vi "Aurdino Mode Lights.vi"(0 "Climb":bool, 7 "Tracks Down":bool, 8 "Robot Centric":bool, 9 "Field Centric":bool) -> ()   [LabVIEW 2017]
uses:
  <vilib>/Rock Robotics/Network Tables/NT Read Boolean.vi
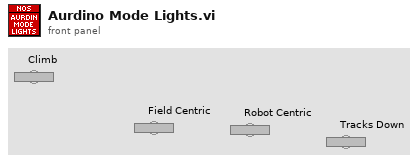
[diagram p1: front panel]
types:
  T1 = typedef "WPI_DigitalInputDevRef.ctl" = cluster{"DevStatus":errorcluster, "DIO Channel":T2}
  T2 = typedef "FPGA_DIOChannel.ctl" = enum8{"DIO 0", "DIO 1", "DIO 2", "DIO 3", "DIO 4", "DIO 5", "DIO 6", "DIO 7", "DIO 8", "DIO 9", "DIO MXP 0", "DIO MXP 1", "DIO MXP 2", "DIO MXP 3", "DIO MXP 4", "DIO MXP 5", "DIO MXP 6", "DIO MXP 7", "DIO MXP 8", "DIO MXP 9", "DIO MXP 10", "DIO MXP 11", "DIO MXP 12", "DIO MXP 13", "DIO MXP 14", "DIO MXP 15", "SPI Port CS1", "SPI Port CS2", "SPI Port CS3", "SPI Port MISO", "SPI Port MOSI", "Invalid"}
  T3 = typedef "WPI_DigitalOutputDevRef.ctl" = cluster{"DIO Channel":T2, "DevStatus":errorcluster}
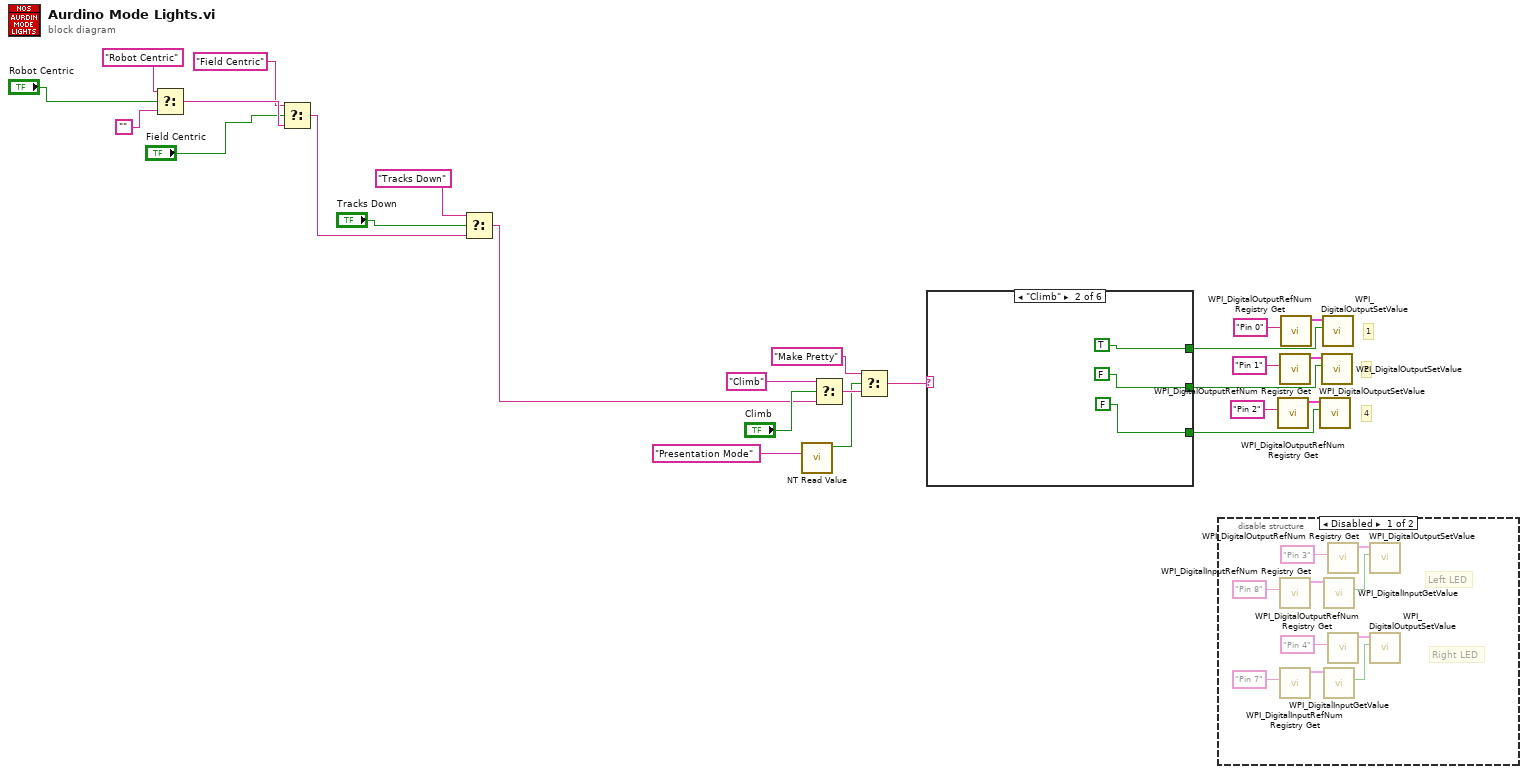
[diagram p0: block diagram]
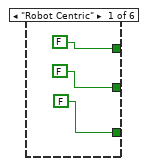
[diagram p3: hidden frame]
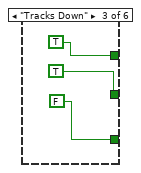
[diagram p4: hidden frame]
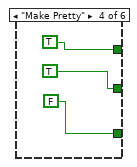
[diagram p5: hidden frame]
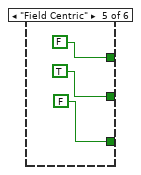
[diagram p6: hidden frame]
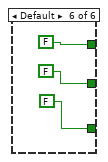
[diagram p7: hidden frame]
diagram:
  # "4"
  # "2"
  # "1"
  n1 = Select(t="Robot Centric", s="Robot Centric", f="") -> (s? t:f=w19:string)
  n2 = Select(t="Field Centric", s="Field Centric", f=w19) -> (s? t:f=w17:string)
  n3 = Select(t="Tracks Down", s="Tracks Down", f=w17) -> (s? t:f=w3:string)
  n4 = call-poly <vilib>:"NT Read Value.vi"("Name"="Presentation Mode") -> ("Boolean"=w2:bool)  [unwired: 9 in, 1 out]
  n5 = Select(t="Climb", s="Climb", f=w3) -> (s? t:f=w11:string)
  n6 = Select(t="Make Pretty", s=w2, f=w11) -> (s? t:f=w12:string)
  n7 = case shown="\"Climb\"" w12 {
    tunnel: [FALSE TRUE TRUE TRUE FALSE FALSE] -> w6
    tunnel: [FALSE FALSE TRUE TRUE TRUE FALSE] -> w7
    tunnel: [FALSE FALSE FALSE FALSE FALSE FALSE] -> w8
    frame "Robot Centric" {
    }
    frame "Climb" {
    }
    frame "Tracks Down" {
    }
    frame "Make Pretty" {
    }
    frame "Field Centric" {
    }
    frame Default {
    }
  }
  n8 = disable-structure shown="Disabled" {
    frame Disabled {
      # "Right LED"
      # "Left LED"
      n9 = call <vilib>:"WPI_DigitalInputRefNum Registry Get.vi"("refnum name"="Pin 8") -> ("DigitalInputDevRef"=w52:T1)  [unwired: 9 in, 1 out]
      n10 = call <vilib>:"WPI_DigitalInputRefNum Registry Get.vi"("refnum name"="Pin 7") -> ("DigitalInputDevRef"=w49:T1)  [unwired: 9 in, 1 out]
      n11 = call <vilib>:"WPI_DigitalInputGetValue.vi"("DigitalInputDevRef"=w52) -> ("Value"=w50:bool)  [unwired: 8 in, 2 out]
      n12 = call <vilib>:"WPI_DigitalInputGetValue.vi"("DigitalInputDevRef"=w49) -> ("Value"=w46:bool)  [unwired: 8 in, 2 out]
      n13 = call <vilib>:"WPI_DigitalOutputRefNum Registry Get.vi"("refnum name"="Pin 3") -> ("DigitalOutputDevRef"=w54:T3)  [unwired: 9 in, 1 out]
      n14 = call <vilib>:"WPI_DigitalOutputRefNum Registry Get.vi"("refnum name"="Pin 4") -> ("DigitalOutputDevRef"=w47:T3)  [unwired: 9 in, 1 out]
      n15 = call <vilib>:"WPI_DigitalOutputSetValue.vi"("Value"=w50, "DigitalOutputDevRef"=w54) -> ()  [unwired: 8 in, 2 out]
      n16 = call <vilib>:"WPI_DigitalOutputSetValue.vi"("Value"=w46, "DigitalOutputDevRef"=w47) -> ()  [unwired: 8 in, 2 out]
    }
    frame Enabled {
    }
  }
  n17 = call <vilib>:"WPI_DigitalOutputRefNum Registry Get.vi"("refnum name"="Pin 2") -> ("DigitalOutputDevRef"=w24:T3)  [unwired: 9 in, 1 out]
  n18 = call <vilib>:"WPI_DigitalOutputRefNum Registry Get.vi"("refnum name"="Pin 1") -> ("DigitalOutputDevRef"=w25:T3)  [unwired: 9 in, 1 out]
  n19 = call <vilib>:"WPI_DigitalOutputRefNum Registry Get.vi"("refnum name"="Pin 0") -> ("DigitalOutputDevRef"=w26:T3)  [unwired: 9 in, 1 out]
  n20 = call <vilib>:"WPI_DigitalOutputSetValue.vi"("Value"=w8, "DigitalOutputDevRef"=w24) -> ()  [unwired: 8 in, 2 out]
  n21 = call <vilib>:"WPI_DigitalOutputSetValue.vi"("Value"=w7, "DigitalOutputDevRef"=w25) -> ()  [unwired: 8 in, 2 out]
  n22 = call <vilib>:"WPI_DigitalOutputSetValue.vi"("Value"=w6, "DigitalOutputDevRef"=w26) -> ()  [unwired: 8 in, 2 out]
